vi "Read write operation timeout.vi"(8 "error in (no error)":errorcluster, 11 "transmission data unit in":refnum<class "Transmission Data Unit.lvclass">) -> (0 "error out":errorcluster, 2 "write operation timeout":i32, 3 "transmission data unit out":refnum<class "Transmission Data Unit.lvclass">)   [LabVIEW 2013, in "Modbus Library - Advance.lvlib" / "Transmission Data Unit.lvclass"]
uses:
  Transmission Data Unit.lvclass
  Transmission Data Unit.lvclass/Transmission Data Unit.ctl
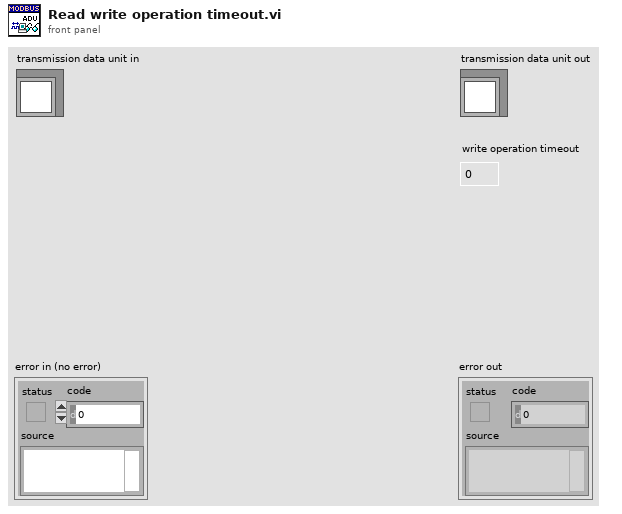
[diagram p1: front panel]
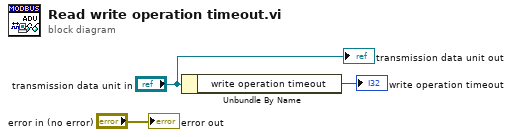
[diagram p0: block diagram]
diagram:
  n1 = Unbundle By Name("transmission data unit in") -> ("write operation timeout"=→"write operation timeout":i32)
  "error out" <- "error in (no error)"
  "transmission data unit out" <- "transmission data unit in"
